vi "ADIS16470 Encode Address.vi"(9 "Data":u16 format="%x", 10 "Address":u16 format="%x") -> (1 "High Word":u8[](array[numeric]), 2 "Low Word":u8[](array[numeric]))   [LabVIEW 2020]
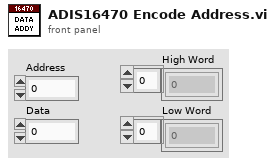
[diagram p1: front panel]
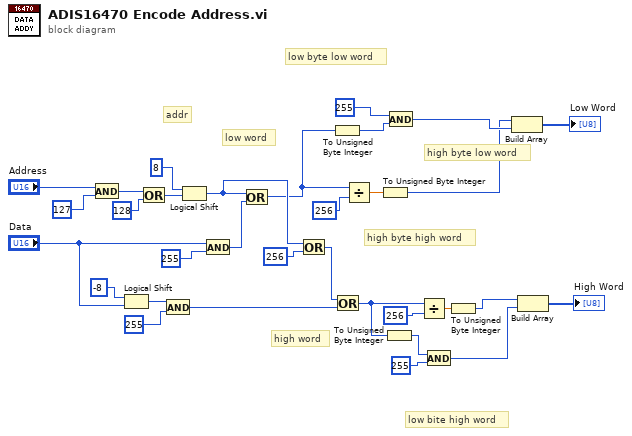
[diagram p0: block diagram]
diagram:
  # "low byte low word"
  # "high byte low word"
  # "low bite high word"
  # "high byte high word"
  # "addr"
  # "high word"
  # "low word"
  n1 = And(x="Address", y=u16 127) -> (x .and. y?=w30:u16)
  n2 = Logical Shift(y=i16 -8, x="Data") -> (x << y=w22:u16)
  n3 = Or(x=w30, y=u16 128) -> (x .or. y?=w28:u16)
  n4 = And(x=w22, y=u16 255) -> (x .and. y?=w20:u16)
  n5 = Logical Shift(y=i16 8, x=w28) -> (x << y=w19:u16)
  n6 = And(x="Data", y=u16 255) -> (x .and. y?=w25:u16)
  n7 = Or(x=w19, y=w25) -> (x .or. y?=w5:u16)
  n8 = Or(x=w19, y=u16 256) -> (x .or. y?=w17:u16)
  n9 = To Unsigned Byte Integer(number=w5) -> (unsigned 8bit integer=w11:u8)
  n10 = Or(x=w17, y=w20) -> (x .or. y?=w10:u16)
  n11 = Divide(x=w5, y=u16 256) -> (x/y=w3:dbl)
  n12 = To Unsigned Byte Integer(number=w3) -> (unsigned 8bit integer=w6:u8)
  n13 = To Unsigned Byte Integer(number=w10) -> (unsigned 8bit integer=w13:u8)
  n14 = And(x=u8 255, y=w11) -> (x .and. y?=w12:u8)
  n15 = Divide(x=w10, y=u16 256) -> (x/y=w8:dbl)
  n16 = And(x=w13, y=u8 255) -> (x .and. y?=w14:u8)
  n17 = To Unsigned Byte Integer(number=w8) -> (unsigned 8bit integer=w7:u8)
  n18 = Build Array(w6, w12) -> (→"Low Word":u8[])
  n19 = Build Array(w7, w14) -> (→"High Word":u8[])
